vi "String to Config.vi"(6 "compatible?":bool, 8 "error in (no error)":errorcluster, 10 "string input":string, 11 "queue in":T1) -> (0 "error out":errorcluster, 3 "queue out":T1)   [LabVIEW 2020, in "NI_LVConfig.lvlib"]
uses:
  <vilib>/Utility/config.llb/NI_LVConfig.lvlib
  <vilib>/Utility/config.llb/Config Queue.ctl
  <vilib>/Utility/config.llb/Config Data.ctl
  <vilib>/Utility/config.llb/Section.ctl
panel:
  out "before substring":string
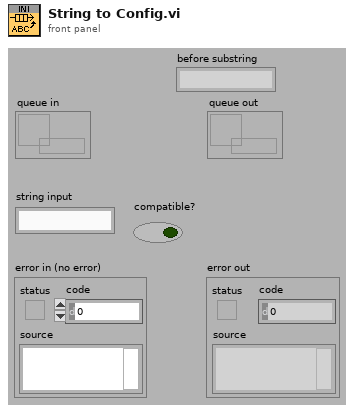
[diagram p1: front panel]
types:
  T1 = typedef "NI_LVConfig.lvlib/Config Queue.ctl" = refnum<queue>
  T2 = typedef "NI_LVConfig.lvlib/Section.ctl" = cluster{"name":string, "comment":string, "kvc":string[][]}
  T3 = typedef "NI_LVConfig.lvlib/Config Data.ctl" = cluster{"sections":T2[], "path":path, "dirty":bool}
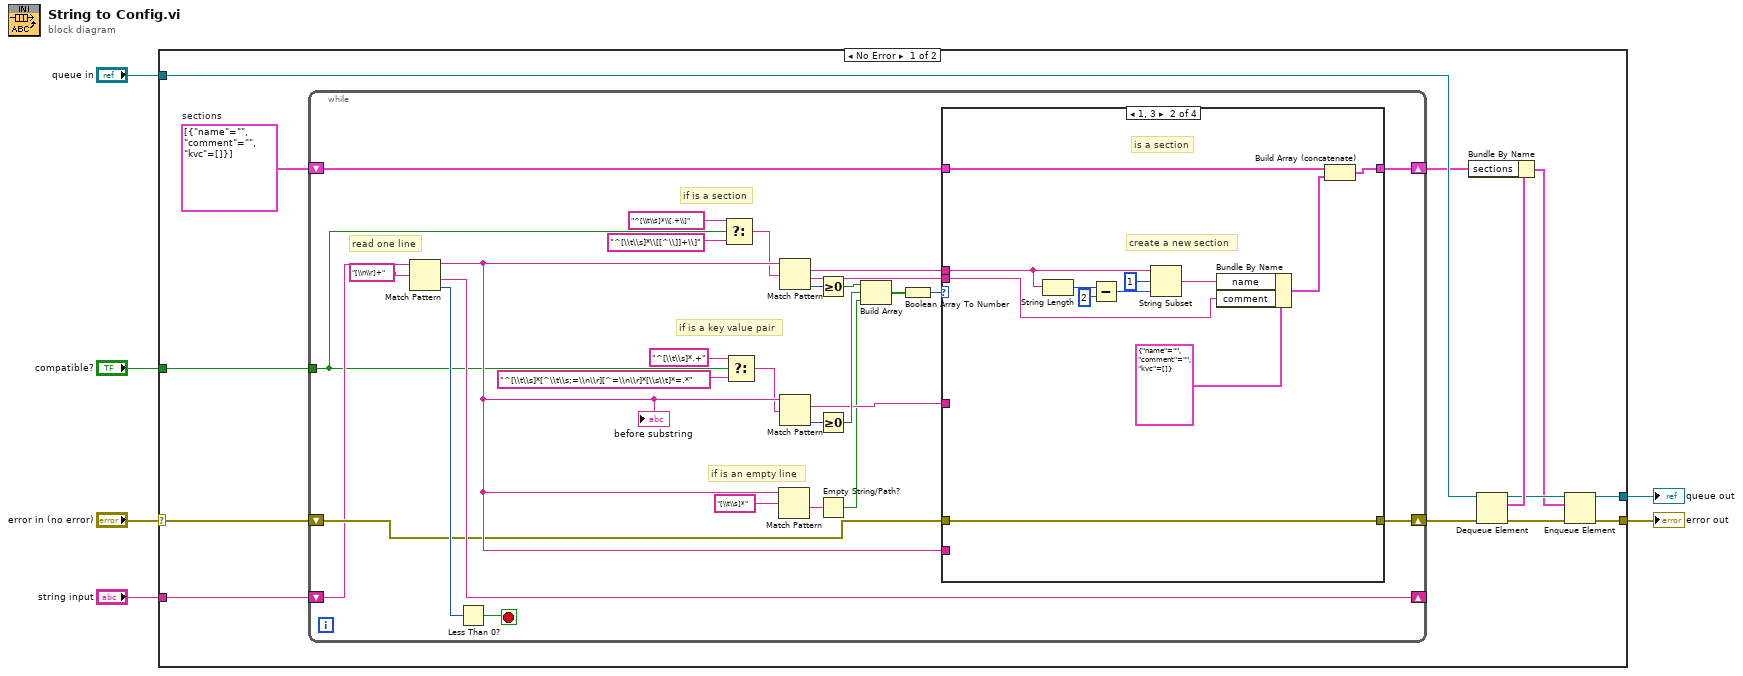
[diagram p0: block diagram]
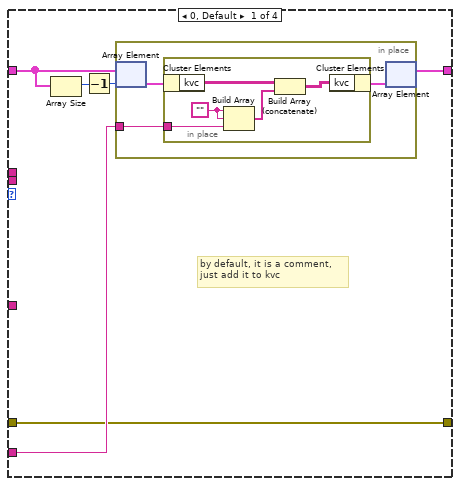
[diagram p2: hidden frame]
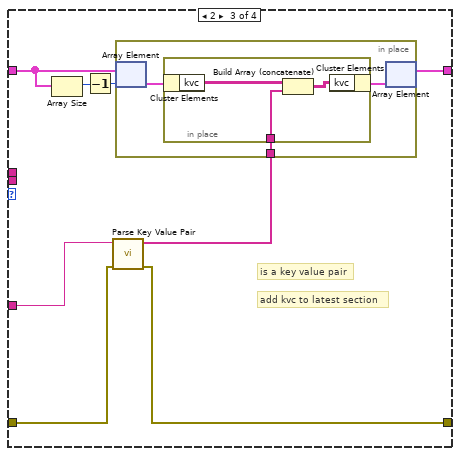
[diagram p3: hidden frame]
diagram:
  n1 = case shown="No Error" "error in (no error)" {
    selector: "error in (no error)" -> [w10 w92]
    tunnel: "queue in" -> [w19 w91]
    tunnel: [w16 w91] -> w3
    tunnel: "string input" -> [w8 _]
    tunnel: [w13 w92] -> w5
    tunnel: "compatible?" -> [w7 _]
    frame No Error {
      w12 = T2[] [{"name"="", "comment"="", "kvc"=[]}]  # sections
      n2 = while {
        shift-right: [w39] -> w11
        shift-left: w12 -> [w40]
        shift-right: [w37] -> w9
        shift-left: w10 -> [w26]
        shift-right: [w33] -> _
        shift-left: w8 -> [w24]
        tunnel: w7 -> [w20]
        stop <- w35 stop-if-true
        # "if is an empty line"
        # "if is a key value pair"
        # "if is a section"
        # "read one line"
        n3 = Match Pattern(string=w24, regular expression="[\\n\\r]+") -> (before substring=w31:string, after substring=w33:string, offset past match=w34:i32)  [unwired: 1 in, 1 out]
        "before substring" <- w31
        n4 = Less Than 0?(x=w34) -> (x < 0?=w35:bool)
        n5 = Select(t="^[\\t\\s]*\\[.+\\]" ("regular expression"), s=w20, f="^[\\t\\s]*\\[[^\\]]+\\]" ("regular expression")) -> (s? t:f=w21:string)
        n6 = Select(t="^[\\t\\s]*.+" ("regular expression"), s=w20, f="^[\\t\\s]*[^\\t\\s;=\\n\\r][^=\\n\\r]*[\\s\\t]*=.*" ("regular expression")) -> (s? t:f=w28:string)
        n7 = Match Pattern(string=w31, regular expression="[\\t\\s]*") -> (after substring=w36:string)  [unwired: 1 in, 3 out]
        n8 = Match Pattern(string=w31, regular expression=w21) -> (match substring=w43:string, after substring=w41:string, offset past match=w48:i32)  [unwired: 1 in, 1 out]
        n9 = Match Pattern(string=w31, regular expression=w28) -> (match substring=w42:string, offset past match=w25:i32)  [unwired: 1 in, 2 out]
        n10 = Greater Or Equal To 0?(x=w48) -> (x >= 0?=w47:bool)
        n11 = Greater Or Equal To 0?(x=w25) -> (x >= 0?=w46:bool)
        n12 = Empty String/Path?(string/path=w36) -> (empty?=w38:bool)
        n13 = Build Array(w47, w46, w38) -> (w45:bool[])
        n14 = Boolean Array To Number(Boolean array=w45) -> (number=w44:u32)
        n15 = case shown="1, 3" w44 {
          tunnel: w43 -> [_ w63 _ _]
          tunnel: w42 -> [_ _ w78 _]
          tunnel: w31 -> [w51 _ _ _]
          tunnel: w41 -> [_ w64 _ _]
          tunnel: w40 -> [w54 w67 w82 w90]
          tunnel: [w50 w66 w79 w90] -> w39
          tunnel: w26 -> [w49 w65 w76 w89]
          tunnel: [w49 w65 w75 w89] -> w37
          frame 0, Default {
            # "by default, it is a comment, \njust add it to kvc"
            n16 = Array Size(array=w54) -> (size(s)=w52:i32)
            n17 = Decrement(x=w52) -> (x-1=w53:i32)
            n18 = in-place {
              in-place-border: w51 -> [w57]
              n19 = in-place-array #1(w54, w53) -> (w56:T2)
              n20 = in-place {
                in-place-border: w57 -> [w61]
                w62 = ""
                n21 = in-place-cluster #2(w56) -> ("kvc"=w59:string[][])
                n22 = Build Array(w62, w62, w61) -> (w60:string[])
                n23 = Build Array (concatenate)(w59, w60) -> (w58:string[][])
                n24 = in-place-cluster #2("kvc"=w58) -> (w55:T2)
              }
              n25 = in-place-array #1(w55) -> (w50:T2[])  [unwired: 1 out]
            }
          }
          frame 1, 3 {
            # "is a section"
            # "create a new section"
            n26 = String Length(string=w63) -> (length=w72:i32)
            n27 = Subtract(x=w72, y=2) -> (x-y=w73:i32)
            n28 = String Subset(string=w63, offset (0)=1, length (rest)=w73) -> (substring=w69:string)
            n29 = Bundle By Name(cluster=T2 {"name"="", "comment"="", "kvc"=[]} ("Section"), "name"=w69, "comment"=w64) -> (w68:T2)
            n30 = Build Array (concatenate)(w67, w68) -> (w66:T2[])
          }
          frame 2 {
            # "is a key value pair"
            # "add kvc to latest section"
            n31 = Array Size(array=w82) -> (size(s)=w80:i32)
            n32 = Decrement(x=w80) -> (x-1=w81:i32)
            n33 = call <vilib>:"Parse Key Value Pair.vi"("error in (no error)"=w76, "key value pair"=w78) -> ("error out"=w75:errorcluster, "KVC"=w77:string[])  [unwired: 2 in, 6 out]
            n34 = in-place {
              in-place-border: w77 -> [w83]
              n35 = in-place-array #3(w82, w81) -> (w85:T2)
              n36 = in-place {
                in-place-border: w83 -> [w86]
                n37 = in-place-cluster #4(w85) -> ("kvc"=w88:string[][])
                n38 = Build Array (concatenate)(w88, w86) -> (w87:string[][])
                n39 = in-place-cluster #4("kvc"=w87) -> (w84:T2)
              }
              n40 = in-place-array #3(w84) -> (w79:T2[])  [unwired: 1 out]
            }
          }
          frame 4 {
            # "empty line"
          }
        }
      }
      n41 = Dequeue Element(queue=w19, error in (no error)=w9) -> (queue out=w17:T1, element=w18:T3, error out=w14:errorcluster)  [unwired: 2 out]
      n42 = Bundle By Name(cluster=w18, "sections"=w11) -> (w15:T3)
      n43 = Enqueue Element(queue=w17, element=w15, error in (no error)=w14) -> (queue out=w16:T1, error out=w13:errorcluster)  [unwired: 2 out]
    }
    frame Error {
    }
  }
  "error out" <- w5
  "queue out" <- w3
